vi "Send_UIWriteCtrl.vi"(5 "Class_Hierarchy (F)":bool, 6 "HighPriority (F)":bool, 7 "Value Signaling (F)":bool, 8 "error in":errorcluster, 9 "Control Data":variant, 10 "Control Label":string, 11 "Queue in":refnum<queue>) -> (0 "error out":errorcluster)   [LabVIEW 2018, in "UI_Library.lvlib"]
uses:
  UI_Library.lvlib
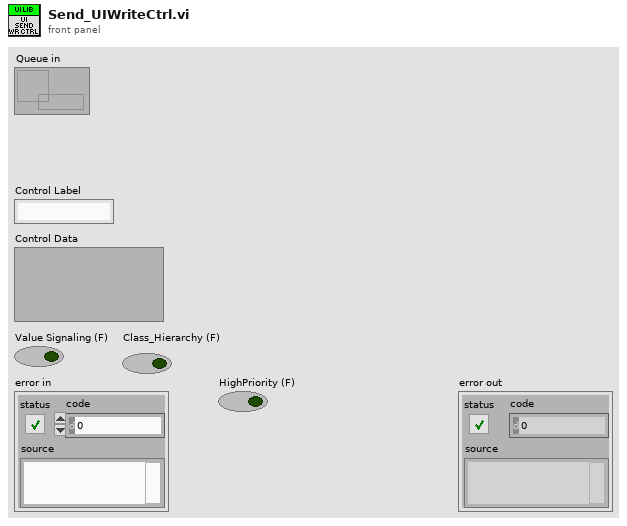
[diagram p1: front panel]
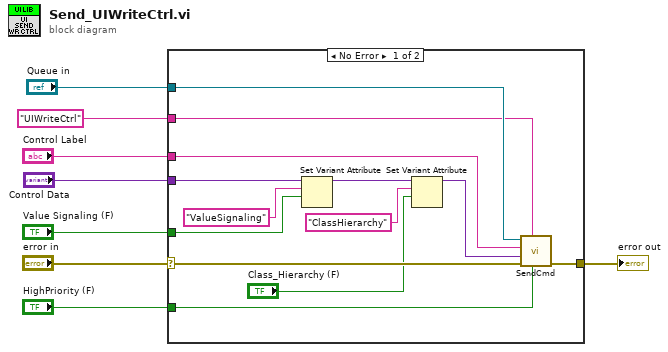
[diagram p0: block diagram]
diagram:
  n1 = case shown="No Error" "error in" {
    selector: "error in" -> [w20 w22]
    tunnel: "Queue in" -> [w21 _]
    tunnel: "Control Label" -> [w17 _]
    tunnel: "Control Data" -> [w14 _]
    tunnel: "UIWriteCtrl" ("UICmd") -> [w18 _]
    tunnel: "HighPriority (F)" -> [w16 _]
    tunnel: [w19 w22] -> w8
    tunnel: "Value Signaling (F)" -> [w13 _]
    frame No Error {
      n2 = Set Variant Attribute(Variant=w14, name="ValueSignaling", value=w13) -> (Variant out=w12:variant)  [unwired: 1 in, 2 out]
      n3 = Set Variant Attribute(Variant=w12, name="ClassHierarchy", value="Class_Hierarchy (F)") -> (Variant out=w11:variant)  [unwired: 1 in, 2 out]
      n4 = call "SendCmd.vi"("HighPriority (F)"=w16, "UICmd"=w18, "error in"=w20, "Control Data"=w11, "Control Label"=w17, "Queue in"=w21) -> ("error out"=w19:errorcluster)  [unwired: 5 in]
    }
    frame Error {
    }
  }
  "error out" <- w8
